vi "VAR_Query.vi"(0 "System no.":i32=1 min=1 max=4 step=1, 2 "Variable name":string[](array[string]), 3 "All Var.?":bool, 5 "error in":errorcluster) -> (14 "Value":string[](array[string]), 19 "error out":errorcluster)   [LabVIEW 2020]
doc: "Returns the value of given variable name(s). See controller user manual for details regarding local and global variables.\n\nC-887, F-206, M-8X0: For GCS syntax version = GCS 2.0 or higher (Check with CSV?.vi. If CSV?.vi is not supported, syntax version is GCS 1.0).\n\nC-867, Mercury_GCS :"
panel:
  # "Returns the value of given variable name(s). See controller User Manual \nfor details regarding local and global variables."
  # "Query"
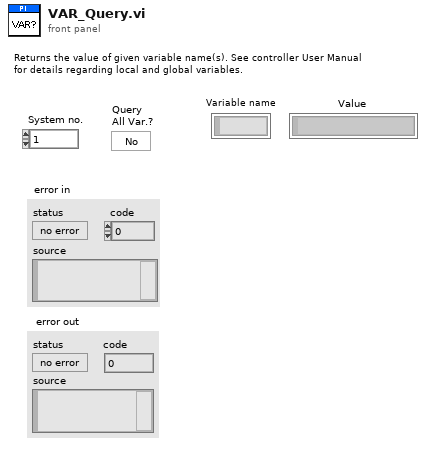
[diagram p1: front panel]
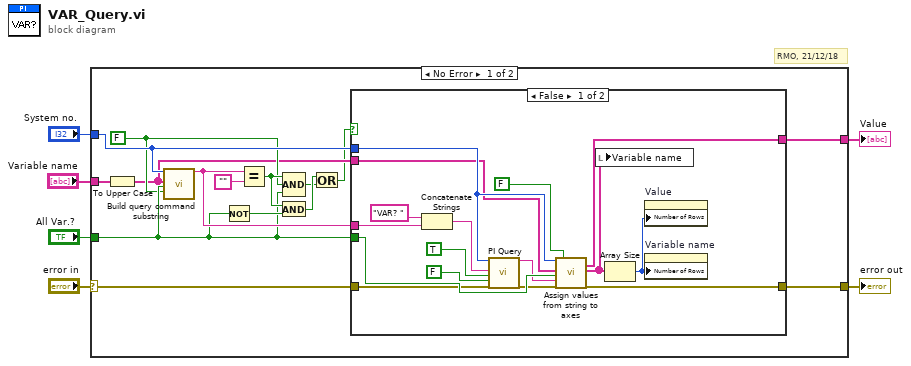
[diagram p0: block diagram]
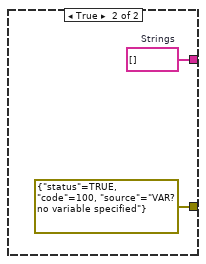
[diagram p2: hidden frame]
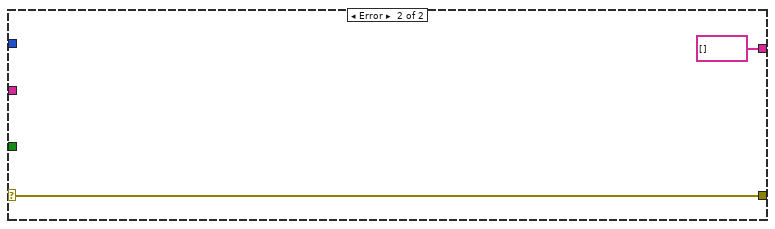
[diagram p3: hidden frame]
diagram:
  # "RMO, 21/12/18"
  n1 = case shown="No Error" "error in" {
    selector: "error in" -> [w9 w40]
    tunnel: "Variable name" -> [w21 _]
    tunnel: [w8 w40] -> w5
    tunnel: "System no." -> [w18 _]
    tunnel: "All Var.?" -> [w14 _]
    tunnel: [w12 string[] [] ("Strings")] -> w2
    frame No Error {
      w11 = FALSE
      n2 = To Upper Case(1:w21) -> (0:w10:string[])
      n3 = call "Build query command substring.vi"("System no."=w18, "Axes to query in"=w10, "Query\nAll axes?"=w14, "For all axes: use\nAxis identifier?"=w11) -> ("Command substring"=w19:string)  [unwired: 2 in, 13 out]
      n4 = Not(x=w14) -> (.not. x?=w17:bool)
      n5 = Equal?(x=w19, y="" ("x")) -> (x = y?=w15:bool)
      n6 = And(x=w15, y=w17) -> (x .and. y?=w16:bool)
      n7 = Compound Arithmetic op=AND(w15, w11, w14) -> (w13:bool)
      n8 = Or(x=w16, y=w13) -> (x .or. y?=w7:bool)
      n9 = case shown="False" w7 {
        tunnel: w19 -> [w34 _]
        tunnel: w18 -> [w33 _]
        tunnel: w14 -> [w32 _]
        tunnel: [w31 w38] -> w12
        tunnel: w10 -> [w28 _]
        tunnel: w9 -> [w26 _]
        tunnel: [w25 errorcluster {"status"=TRUE, "code"=100, "source"="VAR? no variable specified"} ("error out")] -> w8
        frame False {
          n10 = Concatenate Strings("VAR? ", w34) -> (w35:string)
          n11 = call "PI Query.vi"("System no."=w33, "String to send"=w35, "Attach termination char.?"=TRUE ("Attach Linefeed?"), "Strip spaces?"=FALSE, "error in"=w26) -> ("String read"=w23:string, "error out"=w24:errorcluster)  [unwired: 2 in, 11 out]
          n12 = call "Assign values from string to axes.vi"("System no."=w33, "Queried axes"=w28, "All axes queried?"=w32, "Input String"=w23, "error in"=w24, "Axes related?"=FALSE) -> ("Strings"=w31:string[], "Queried axes out"=w29:string[], "error out"=w25:errorcluster)  [unwired: 3 in, 8 out]
          n13 = local write "Variable name"(w29) -> ()
          n14 = Array Size(array=w29) -> (size(s)=w30:i32)
          n15 = property on="Value" class="Arr (strict)"("Number of Rows"=w30) -> ()  [unwired: 2 in, 2 out]
          n16 = property on="Variable name" class="Arr (strict)"("Number of Rows"=w30) -> ()  [unwired: 2 in, 2 out]
        }
        frame True {
          w38 = string[] []  # Strings
        }
      }
    }
    frame Error {
    }
  }
  "error out" <- w5
  "Value" <- w2
